vi "Misc.vi"() -> ()   [LabVIEW 2018]
panel:
  in  "Boolean":bool=TRUE
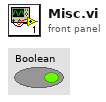
[diagram p1: front panel]
types:
  T1 = typedef "WPI_CompressorDevRef.ctl" = cluster{"DevStatus":errorcluster, "Pneumatics Control Module":u8}
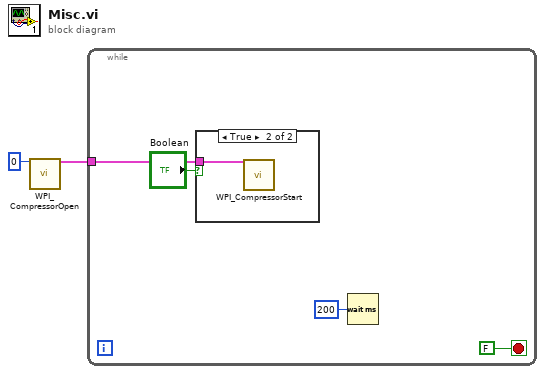
[diagram p0: block diagram]
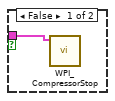
[diagram p2: hidden frame]
diagram:
  n1 = call <vilib>:"WPI_CompressorOpen.vi"("Pneumatics Control Module (0)"=u8 0) -> ("CompressorDevRef"=w1:T1)  [unwired: 13 in, 1 out]
  n2 = while {
    tunnel: w1 -> [w5]
    stop <- FALSE stop-if-true
    n3 = case shown="True" "Boolean" {
      tunnel: w5 -> [w7 w8]
      frame False {
        n4 = call <vilib>:"WPI_CompressorStop.vi"("CompressorDevRef"=w7) -> ()  [unwired: 9 in, 2 out]
      }
      frame True {
        n5 = call <vilib>:"WPI_CompressorStart.vi"("CompressorDevRef"=w8) -> ()  [unwired: 9 in, 2 out]
      }
    }
    n6 = Wait (ms)(milliseconds to wait=u32 200) -> ()  [unwired: 1 out]
  }
